vi "process.vi"(8 "error in":errorcluster, 9 "result allocation":T1, 10 "parameters":T1, 11 "module in":refnum<class "Tagbus PID Module runtime.lvclass">) -> (0 "error out":errorcluster, 1 "results":T1, 2 "parameter allocation":T1, 3 "module out":refnum<class "Tagbus PID Module runtime.lvclass">)   [LabVIEW 2014, in "Tagbus PID Module runtime.lvclass"]
doc: "Provides an interface for information processing by a module at runtime. While this interface performs no operations, a child should provide an override which may process data in any manner necessary."
uses:
  Tagbus PID Module runtime.lvclass
  <vilib>/NI/Tag Bus/table/data table.ctl
  Tagbus PID Module runtime.lvclass/Tagbus PID Module runtime.ctl
  <vilib>/addons/control/pid/pid.llb/PID (DBL Array).vi
  <vilib>/NI/Tag Bus Module Framework/runtime/TBM module execution interface.lvclass
  <vilib>/addons/control/pid/NI_PID_pid.lvlib
  <vilib>/NI/Tag Bus/table/data table.lvlib
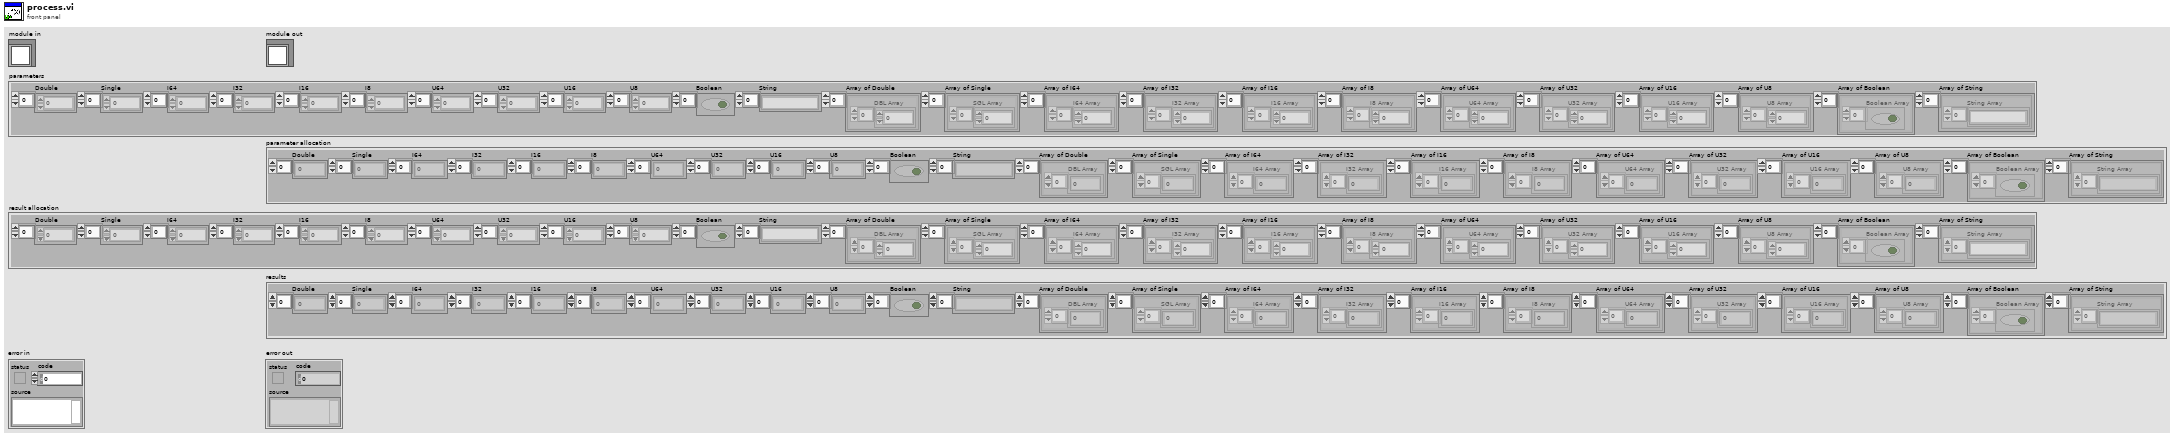
[diagram p1: front panel]
types:
  T1 = typedef "tag bus.lvlib/data table.lvlib/data table.ctl" = cluster{"Double":dbl[], "Single":sgl[], "I64":i64[], "I32":i32[], "I16":i16[], "I8":i8[], "U64":u64[], "U32":u32[], "U16":u16[], "U8":u8[], "Boolean":bool[], "String":string[], "Array of Double":cluster{"DBL Array":dbl[]}[], "Array of Single":cluster{"SGL Array":sgl[]}[], "Array of I64":cluster{"I64 Array":i64[]}[], "Array of I32":cluster{"I32 Array":i32[]}[], "Array of I16":cluster{"I16 Array":i16[]}[], "Array of I8":cluster{"I8 Array":i8[]}[], "Array of U64":cluster{"U64 Array":u64[]}[], "Array of U32":cluster{"U32 Array":u32[]}[], "Array of U16":cluster{"U16 Array":u16[]}[], "Array of U8":cluster{"U8 Array":u8[]}[], "Array of Boolean":cluster{"Boolean Array":bool[]}[], "Array of String":cluster{"String Array":string[]}[]}
  T2 = typedef "Tagbus PID Module runtime.lvclass/processing inputs.ctl" = cluster{"Setpoints":i32[], "Process Variables":i32[], "Gains":cluster{"proportional gain (Kc)":dbl, "integral time (Ti, min)":dbl, "derivative time (Td, min)":dbl}[], "Range":cluster{"output high":dbl, "output low":dbl}[]}
  T3 = typedef "Tagbus PID Module runtime.lvclass/processing outputs.ctl" = cluster{"Outputs":i32[]}
  T4 = cluster{"proportional gain (Kc)":dbl, "integral time (Ti, min)":dbl, "derivative time (Td, min)":dbl}[]
  T5 = cluster{"Setpoints":dbl[], "Process Variables":dbl[]}
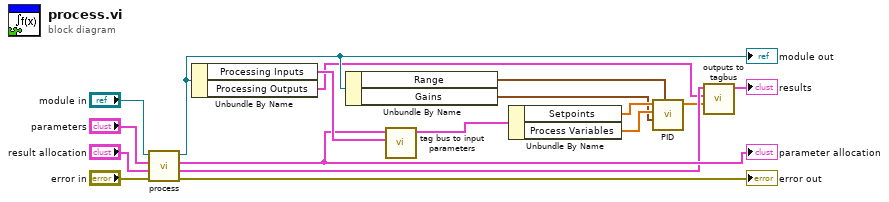
[diagram p0: block diagram]
diagram:
  n1 = call-parent "process.vi"("error in"="error in", "result allocation"="result allocation", "parameters"="parameters", "module in"="module in") -> ("error out"=→"error out":errorcluster, "results"=w5:T1, "parameter allocation"=w11:T1, "module out"=w2:refnum<class "Tagbus PID Module runtime.lvclass">)  [unwired: 4 in]
  "module out" <- w2
  "parameter allocation" <- w11
  n2 = Unbundle By Name(w2) -> ("Processing Inputs"=w12:T2, "Processing Outputs"=w1:T3)
  n3 = Unbundle By Name(w2) -> ("Range"=w6:cluster{"output high":dbl, "output low":dbl}[], "Gains"=w7:T4)
  n4 = call "tag bus to input parameters.vi"("Processing Inputs"=w12, "parameter allocation"=w11) -> ("inputs"=w10:T5)  [unwired: 9 in]
  n5 = Unbundle By Name(w10) -> ("Setpoints"=w9:dbl[], "Process Variables"=w8:dbl[])
  n6 = call-poly <vilib>:"PID.vi"("output range"=w6, "PID gains"=w7, "process variable"=w8, "setpoint"=w9) -> ("output"=w4:dbl[])  [unwired: 6 in, 1 out]
  n7 = call "outputs to tagbus.vi"("output in"=w4, "Processing Outputs"=w1, "tag bus in"=w5) -> ("tag bus out"=→"results":T1)  [unwired: 8 in]
